vi "Test View Closed on Stop.vi"(8 "error in (no error)":errorcluster, 11 "View Test In":refnum<class "View Test.lvclass">) -> (0 "error out":errorcluster, 3 "View Test Out":refnum<class "View Test.lvclass">)   [LabVIEW 2020, in "View Test.lvclass"]
uses:
  View Test.lvclass
  C:/Program Files (x86)/National Instruments/LabVIEW 2020/vi.lib/Astemes/LUnit/Test Case.lvclass
  Framework/Process/Process.lvclass/Process.ctl
  Framework/View/View.lvclass/View.ctl
  <vilib>/Astemes/LUnit/Test Case.lvclass/Test Case.ctl
  Framework/Process/Protected/Messaging/Request Message.vi
  Framework/Process/Public/Lifecycle/Get Lifecycle State.vi
  Framework/Process/Private/SubVIs/Wait for finish.vi
  Framework/Process/Private/SubVIs/Set Lifecycle State.vi
  Framework/Process/Protected/Messaging/Send Message.vi
  <vilib>/Astemes/LUnit/Set Assertion Type.vi
  <vilib>/Astemes/LUnit/Palette/Pass.vi
  <vilib>/Astemes/LUnit/Palette/Fail.vi
  Framework/Process/Private/SubVIs/Handle Debug Data.vi
  Framework/Process/Private/SubVIs/Enqueue Request Message.vi
  <vilib>/Astemes/LUnit/Add test result.vi
  Framework/Logging/Log Debug.vi
  <vilib>/AdvancedString/1D String Array to Delimited String.vi
  <vilib>/Utility/High Resolution Relative Seconds.vi
  <vilib>/Astemes/LUnit/LUnit Record Assertion Result.vi
  <vilib>/Astemes/LUnit/LUnit Aggregate Assertion Results.vi
  <vilib>/Astemes/LUnit/Method Result/LUnit Merge Status.vi
  <vilib>/Astemes/LUnit/LUnit Concatenate result strings.vi
  Framework/View/View.lvclass
  C:/Git/astemes-triarc-framework/source/Framework/Process/Process.lvclass
  <vilib>/Utility/error.llb/Error Cluster From Error Code.vi
  Framework/Process/Public/Read Name.vi
  Framework/Process/Private/SubVIs/Wait for Response Message.vi
  Framework/Process/Process.lvclass
  View Test.lvclass/View Test.ctl
  C:/Git/astemes-triarc-framework/source/Framework/Base/Base.lvclass
  C:/Git/astemes-triarc-framework/source/Framework/Error Handler Interface/Error Handler Interface.lvclass
  C:/Git/astemes-triarc-framework/source/Framework/Logging/Logging.lvclass
  C:/Git/astemes-triarc-framework/source/Framework/View/View.lvclass
  <vilib>/Astemes/LUnit/Test Case.lvclass
  C:/Git/astemes-triarc-framework/source/Framework Test Suite/Process Test/Process Test.lvclass
  C:/Git/astemes-triarc-framework/source/Framework Test Suite/Base Class Test/Base Test.lvclass
  C:/Git/astemes-triarc-framework/source/Framework Test Suite/View Test/View Test.lvclass
  Process Test/Process Test.lvclass
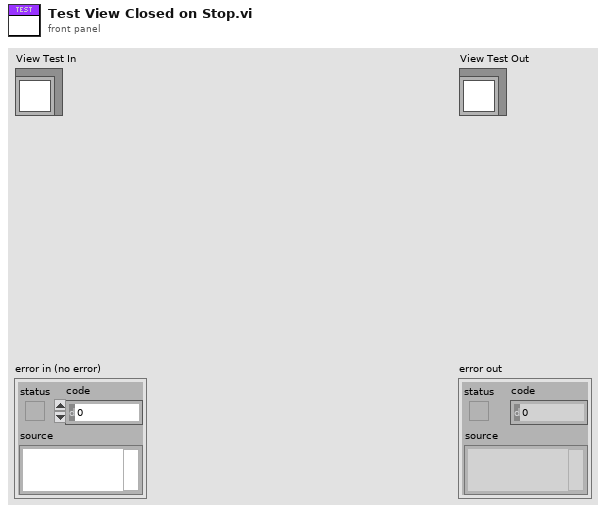
[diagram p1: front panel]
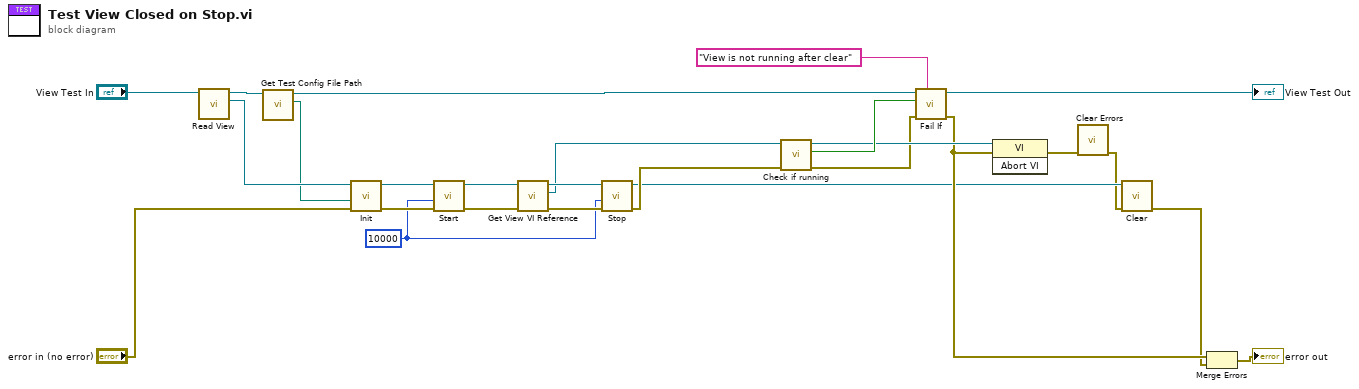
[diagram p0: block diagram]
diagram:
  w14 = 10000 ("Timeout [ms] (-1)")
  n1 = call "Read View.vi"("View Test In"="View Test In") -> ("View"=w25:refnum<class "View.lvclass">, "View Test Out"=w26:refnum<class "View Test.lvclass">)  [unwired: 8 in, 1 out]
  n2 = call "Get Test Config File Path.vi"("Process Test In"=w26) -> ("Test config path"=w1:path, "Process Test Out"=w2:refnum<class "View Test.lvclass">)  [unwired: 8 in, 1 out]
  n3 = call-dynamic "Init.vi"("error in (no error)"="error in (no error)", "Config File Path"=w1, "View In"=w25) -> ("error out"=w19:errorcluster, "View Out"=w20:refnum<class "View.lvclass">)  [unwired: 7 in]
  n4 = call "Start.vi"("error in (no error)"=w19, "Timeout [ms] (-1)"=w14, "Process In"=w20) -> ("error out"=w12:errorcluster, "Process Out"=w13:refnum<class "View.lvclass">)  [unwired: 6 in, 1 out]
  n5 = call "Get View VI Reference.vi"("error in (no error)"=w12, "View In"=w13) -> ("error out"=w17:errorcluster, "View VI Reference"=w16:refnum<vi>, "View Out"=w18:refnum<class "View.lvclass">)  [unwired: 7 in]
  n6 = call "Stop.vi"("error in (no error)"=w17, "timeout in ms (-1)"=w14, "Process In"=w18) -> ("error out"=w15:errorcluster, "Process Out"=w7:refnum<class "View.lvclass">)  [unwired: 6 in, 1 out]
  n7 = call "Check if running.vi"("error in (no error)"=w15, "VI in"=w16) -> ("error out"=w9:errorcluster, "Running?"=w11:bool, "VI out"=w10:refnum<vi>)  [unwired: 7 in]
  n8 = call <vilib>:"Fail If.vi"("Description"="View is not running after clear", "error in (no error)"=w9, "Fail?"=w11, "LUnit Test Case In"=w2) -> ("error out"=w8:errorcluster, "LUnit Test Case Out"=→"View Test Out":refnum<class "View Test.lvclass">)  [unwired: 6 in]
  n9 = invoke class="VI" method="Abort VI"(reference=w10, error in=w8) -> (error out=w6:errorcluster)  [unwired: 1 in, 2 out]
  n10 = call <vilib>:"Clear Errors.vi"("error in (no error)"=w6) -> ("error out"=w5:errorcluster)  [unwired: 5 in, 1 out]
  n11 = call-dynamic "Clear.vi"("error in (no error)"=w5, "View In"=w7) -> ("error out"=w3:errorcluster)  [unwired: 9 in]
  n12 = Merge Errors(w8, w3) -> (→"error out":errorcluster)
